vi "Create Evaluations.vi"(8 "error in (no error)":errorcluster, 11 "IEvaluation in":refnum<class "RxBN dBmHz Calculation.lvclass">) -> (0 "error out":errorcluster, 2 "Evaluations Out":T1[](array[typedef]) {"Low Limit" format="%#_13g"; "SI Scaling" items=["femto"=-15, "pico"=-12, "nano"=-9, "micro"=-6, "milli"=-3, "percent"=-2, ""=0, "kilo"=3, "mega"=6, "giga"=9, "tera"=12]}, 3 "IEvaluation out":refnum<class "RxBN dBmHz Calculation.lvclass">)   [LabVIEW 2016, in "SeqAuto Evaluations.lvlib" / "RxBN dBmHz Calculation.lvclass"]
uses:
  RxBN dBmHz Calculation.lvclass
  C:/projects/STS/Common/Sequence Automation/Plugins/SeqAuto IEvaluation.lvlibp/SeqAuto IEvaluation.lvclass
  Plugins/TestStand API Tools (TSAT).lvlibp/Evaluation Actions/Includes/Controls/TSAT Evaluation.ctl
  Plugins/TestStand API Tools (TSAT).lvlibp/Evaluation Actions/Includes/Controls/TSAT Eval SI Unit Scaling.ctl
  Plugins/TestStand API Tools (TSAT).lvlibp/Evaluation Actions/Includes/Controls/TSAT Evaluation Type.ctl
  RxBN dBmHz Calculation.lvclass/RxBN dBmHz Calculation.ctl
  Read Export Data Locations.vi
  Read Span.vi
  Plugins/SeqAuto IEvaluation.lvlibp/Read Measurement Name.vi
  Plugins/TestStand API Tools (TSAT).lvlibp/Evaluation Actions/TSAT Evaluation Actions.lvlib
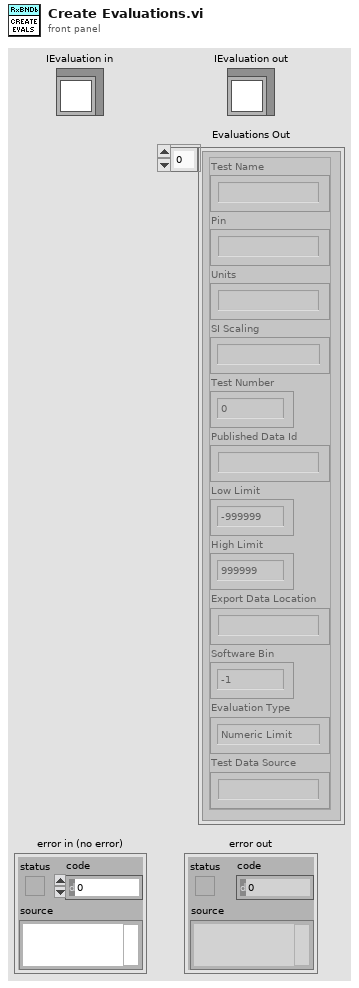
[diagram p1: front panel]
types:
  T1 = typedef "TestStand API Tools (TSAT).lvlibp/TSAT Evaluation Actions.lvlib/TSAT Evaluation.ctl" = cluster{"Test Name":string, "Pin":string, "Units":string, "SI Scaling":T2, "Test Number":i32, "Published Data Id":string, "Low Limit":dbl, "High Limit":dbl, "Export Data Location":string, "Software Bin":i64, "Evaluation Type":T3, "Test Data Source":string}
  T2 = typedef "TestStand API Tools (TSAT).lvlibp/TSAT Evaluation Actions.lvlib/TSAT Eval SI Unit Scaling.ctl" = i16
  T3 = typedef "TestStand API Tools (TSAT).lvlibp/TSAT Evaluation Actions.lvlib/TSAT Evaluation Type.ctl" = enum16{"Numeric Limit", "Pass/Fail", "None"}
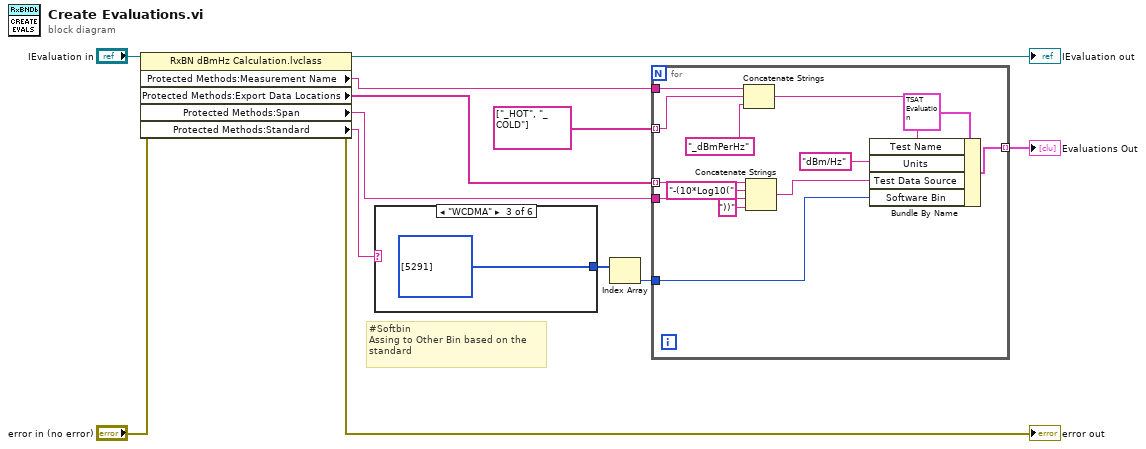
[diagram p0: block diagram]
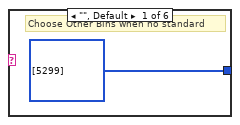
[diagram p2: hidden frame]
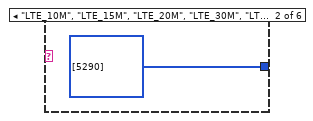
[diagram p3: hidden frame]
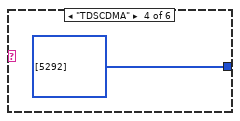
[diagram p4: hidden frame]
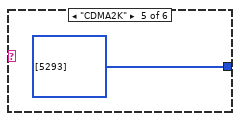
[diagram p5: hidden frame]
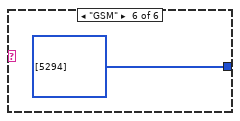
[diagram p6: hidden frame]
diagram:
  # "#Softbin\nAssing to Other Bin based on the \nstandard"
  n1 = property class="RxBN dBmHz Calculation.lvclass"(reference="IEvaluation in", error in="error in (no error)") -> (reference out=→"IEvaluation out":refnum<class "RxBN dBmHz Calculation.lvclass">, error out=→"error out":errorcluster, "Protected Methods:Measurement Name"=w6:string, "Protected Methods:Export Data Locations"=w7:string[], "Protected Methods:Span"=w5:string, "Protected Methods:Standard"=w2:string)
  n2 = case shown="\"WCDMA\"" w2 {
    tunnel: [i64[] [5299] i64[] [5290] i64[] [5291] i64[] [5292] i64[] [5293] i64[] [5294]] -> w3
    frame "", Default {
      # "Choose Other Bins when no standard"
    }
    frame "LTE_10M", "LTE_15M", "LTE_20M", "LTE_30M", "LTE_40M" {
    }
    frame "WCDMA" {
    }
    frame "TDSCDMA" {
    }
    frame "CDMA2K" {
    }
    frame "GSM" {
    }
  }
  n3 = Index Array(array=w3) -> (element=w1:i64)  [unwired: 1 in]
  n4 = for {
    tunnel: [w30] -> w8 mode=indexing
    tunnel: w7 -> [w28] mode=indexing
    tunnel: w6 -> [w26]
    tunnel: w5 -> [w22]
    tunnel: string[] ["_HOT", "_COLD"] -> [w20] mode=indexing
    tunnel: w1 -> [w19]
    n5 = Concatenate Strings(w26, w20, "_dBmPerHz" ("string")) -> (w25:string)
    n6 = Concatenate Strings(w28, "-(10*Log10(" ("string"), w22, "))" ("string")) -> (w27:string)
    n7 = Bundle By Name(cluster=T1 {"Test Name"="", "Pin"="", "Units"="", "SI Scaling"=0, "Test Number"=0, "Published Data Id"="", "Low Limit"=-999999.0, "High Limit"=999999.0, "Export Data Location"="", "Software Bin"=-1, "Evaluation Type"=enum."Numeric Limit", "Test Data Source"=""} ("Evaluation"), "Test Name"=w25, "Units"="dBm/Hz", "Test Data Source"=w27, "Software Bin"=w19) -> (w30:T1)
  }
  "Evaluations Out" <- w8
